vi "Database.SaveResults2.vi"(7 "Idx":i32, 8 "error in (no error)":errorcluster, 9 "Sets":T1, 10 "Data to export":T2, 11 "dbHandle":i32) -> (0 "error out":errorcluster, 1 "Export Time":timestamp, 2 "Data exported":T2, 3 "dbHandle out":i32)   [LabVIEW 2016]
uses:
  Cache/Cache.TestSteps.Fglb.ResultData.ctl
  ProdaNG/Controls/ProdaNG.ProcessResult.ctl
  ProdaNG/Controls/ProdaNG.ProcessStepResult.ctl
  ProdaNG/Controls/ProdaNG.TestStepResult.ctl
  ProdaNG/Controls/ProdaNG.TestValueResult.ctl
  Database.Data.Sets.ctl
  Tools/Translator/Translator.Message.ctl
  Tools/EventLog/EventLog.EventSource.ctl
  ProdaNG/Controls/ProdaNG.Product.ctl
  Tools/EventLog/EventLog.New(array).vi
  Tools/EventLog/EventLog.File.ReadWrite.vi
  Tools/EventLog/EventLog.Buffer.vi
  Global/ApplicationGlobal.vi
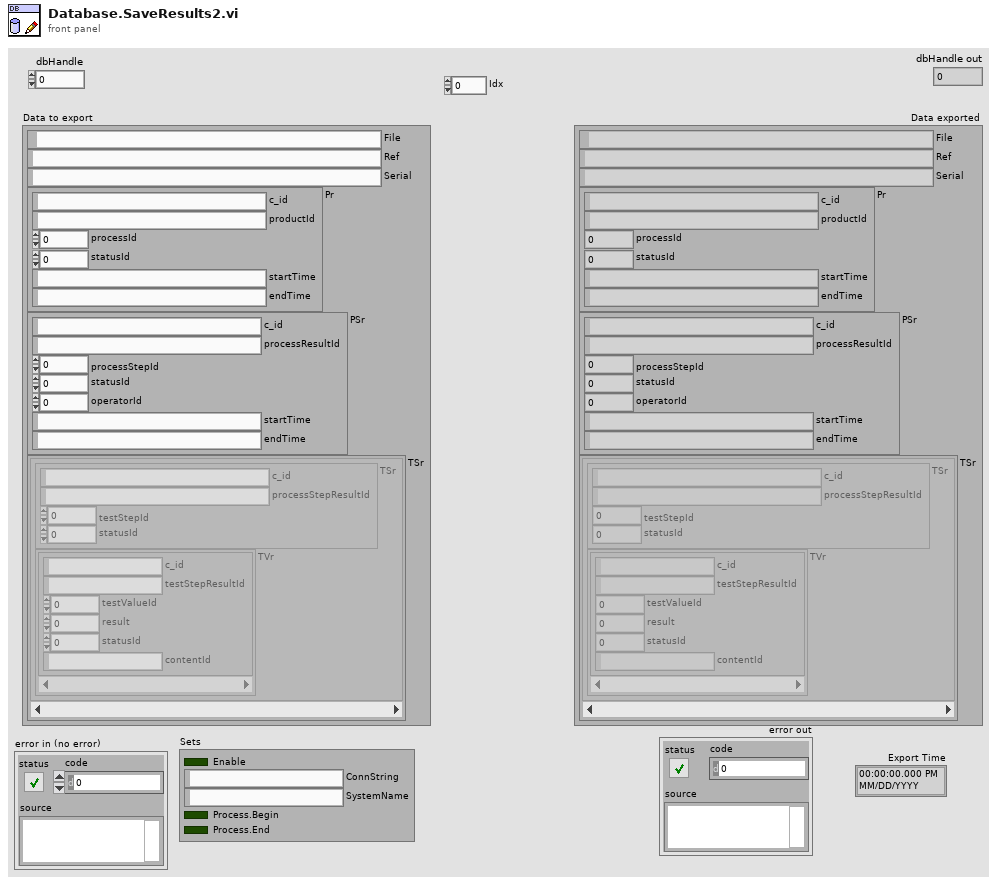
[diagram p1: front panel]
types:
  T1 = typedef "Database.Data.Sets.ctl" = cluster{"Enable":bool, "ConnString":string, "SystemName":string, "Process.Begin":bool, "Process.End":bool}
  T2 = typedef "Cache.TestSteps.Fglb.ResultData.ctl" = cluster{"File":path, "Ref":string, "Serial":string, "Pr":T3, "PSr":T4, "TSr":cluster{"TSr":T5, "TVr":T6[]}[]}
  T3 = typedef "ProdaNG.ProcessResult.ctl" = cluster{"c_id":string, "productId":string, "processId":i32, "statusId":i32, "startTime":string, "endTime":string}
  T4 = typedef "ProdaNG.ProcessStepResult.ctl" = cluster{"c_id":string, "processResultId":string, "processStepId":i32, "statusId":i32, "operatorId":i32, "startTime":string, "endTime":string}
  T5 = typedef "ProdaNG.TestStepResult.ctl" = cluster{"c_id":string, "processStepResultId":string, "testStepId":i32, "statusId":i32}
  T6 = typedef "ProdaNG.TestValueResult.ctl" = cluster{"c_id":string, "testStepResultId":string, "testValueId":i32, "result":dbl, "statusId":i32, "contentId":string}
  T7 = typedef "EventLog.EventSource.ctl" = enum16{"All", "Gui", "Cache", "PLC1", "PLC2", "PLC3", "DB", "DB01", "DB02", "DB03", "DB04", "DB05", "DB06", "DB07", "DB08", "DB09", "DB10", "DB11", "DB12", "DB13", "DB14", "DB15", "DB16"}
  T8 = typedef "Translator.Message.ctl" = enum16{"-", "Event confirmed", "Log out", "Log in", "Shutdown", "Cancel", "Start", "Continue", "Stop", "On", "Off", "OK", "NOK", "NOK %s", "This", "Prev", "Home", "Work", "In progress...", "Missing", "Empty", "Hardware failure", "Initial", "Error %d >> %s", "Error %d >> %s >> %s", "Starting %s", "Quitting %s", "Configured", "Initializing", "Quitting", "Loading", "Running %s", "Stopped", "Summary", "Do you want to continue?", "Do you want to exit?", "Log out?", "System", "All", "IDLE", "Translating...%s", "Not found", "Alarm %s", "Run", "Skip", "Abort", "Repeat", "Please wait...", "Database disconnected", "Login to database successful", "Login to database failed: %d; %s", "Get process step data for %s", "Changeover off", "Changeover into %s", "Product %s | %s found in cache with status %d at previous station", "Product %s | %s found in database with status %d at previous station", "Product %s | %s not found in cache at previous station", "Product %s | %s not found in database at previous station", "Product %s | %s found in cache with status %d at this station (%d repetion)", "Product %s | %s found in database with status %d at this station (%d repetition)", "Product %s | %s not found in cache at this station", "Product %s | %s not found in database at this station", "Product %s | %s found in cache for component %s | %s", "Product %s | %s found in database for component %s | %s", "Product not found in cache for component %s | %s", "Product not found in database for component %s | %s", "Product %s | %s connected with component %s | %s (cache)", "Product %s | %s connected with component %s | %s (database)", "New data for %s | %s (cache)", "New data for %s | %s (database)", "File %s moved (cache)", "File %s deleted (cache)", "Msg %d >> %s", "PLC LifeBit Failure", "Reconnecting DB", "Reconnecting PLC", "Free disk space is below 1GB - contact technician"}
  T9 = typedef "ProdaNG.Product.ctl" = cluster{"c_id":string, "wabcoPartId":i32, "serialNumber":string, "comment":string, "individual":i32, "crProcessStepId":i32, "mdProcessStepId":i32, "crTime":string, "mdTime":string}
  T10 = typedef "ProdaNG.Identification.ctl" = cluster{"processId":i32, "systemId":i32, "processStepId":i32, "wabcoPartId":i32}
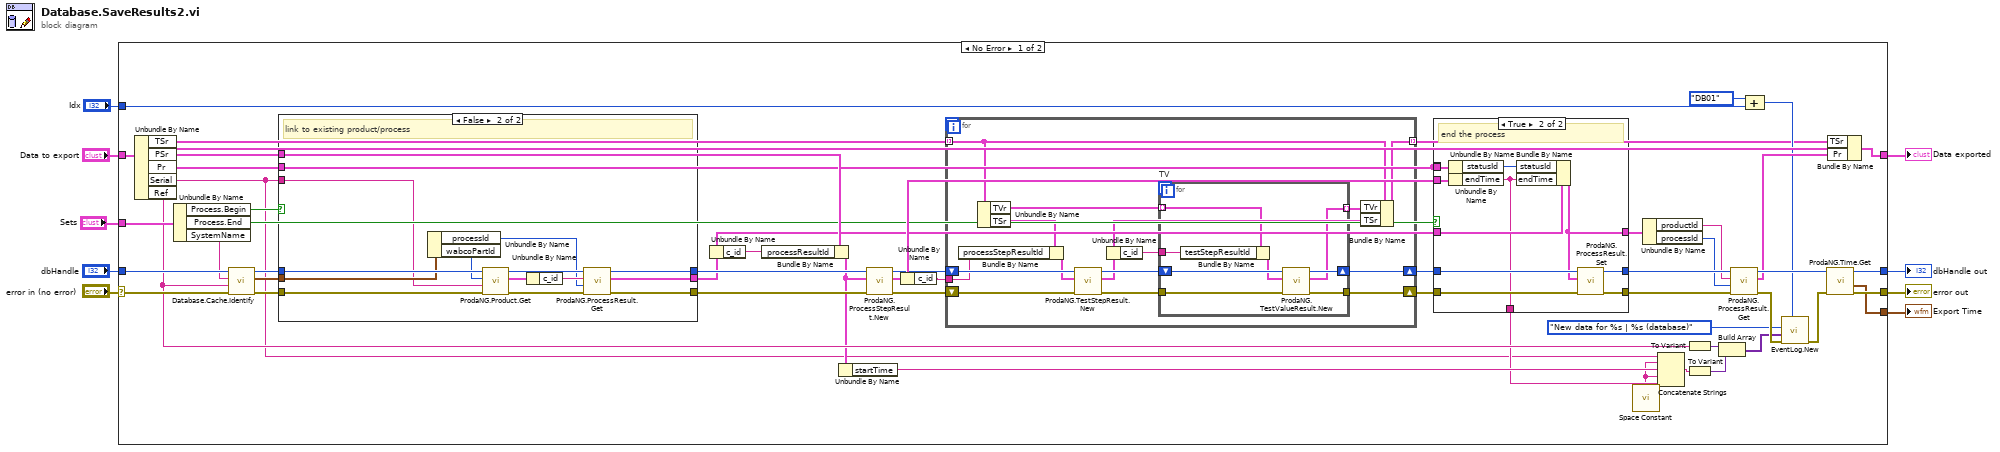
[diagram p0: block diagram]
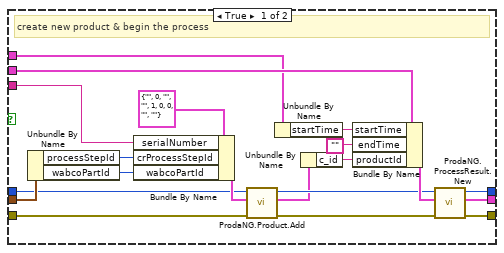
[diagram p2: hidden frame]
diagram:
  n1 = case shown="No Error" "error in (no error)" {
    selector: "error in (no error)" -> [w38 w132]
    tunnel: [w59 w132] -> w9
    tunnel: [w58 w131] -> w7
    tunnel: "dbHandle" -> [w37 w131]
    tunnel: [w57 _] -> w5
    tunnel: "Data to export" -> [w42 w130]
    tunnel: [w43 w130] -> w3
    tunnel: "Sets" -> [w40 _]
    tunnel: "Idx" -> [w30 _]
    frame No Error {
      n2 = Unbundle By Name(w42) -> ("TSr"=w28:cluster{"TSr":T5, "TVr":T6[]}[], "PSr"=w41:T4, "Pr"=w10:T3, "Serial"=w13:string, "Ref"=w29:string)
      n3 = Unbundle By Name(w40) -> ("Process.Begin"=w39:bool, "Process.End"=w25:bool, "SystemName"=w36:string)
      n4 = call "Database.Cache.Identify.vi"("error in (no error)"=w38, "Variant"=w29, "SystemName"=w36, "DB Handle in"=w37) -> ("error out"=w15:errorcluster, "SytemID"=w16:T10, "DB Handle out"=w14:i32)  [unwired: 5 in]
      n5 = case shown="False" w39 {
        tunnel: w14 -> [w90 w112]
        tunnel: w15 -> [w91 w110]
        tunnel: w10 -> [w103 _]
        tunnel: [w101 w116] -> w55
        tunnel: [w100 w114] -> w56
        tunnel: [w99 w115] -> w12
        tunnel: w41 -> [w95 _]
        tunnel: w16 -> [w92 w107]
        tunnel: w13 -> [w84 w104]
        frame True {
          # "create new product & begin the process"
          n6 = Unbundle By Name(w92) -> ("processStepId"=w86:i32, "wabcoPartId"=w85:i32)
          n7 = Bundle By Name(cluster=T9 {"c_id"="", "wabcoPartId"=0, "serialNumber"="", "comment"="", "individual"=1, "crProcessStepId"=0, "mdProcessStepId"=0, "crTime"="", "mdTime"=""} ("Product"), "serialNumber"=w84, "crProcessStepId"=w86, "wabcoPartId"=w85) -> (w93:T9)
          n8 = call "ProdaNG.Product.Add.vi"("error in (no error)"=w91, "Product"=w93, "dbHandle"=w90) -> ("error out"=w88:errorcluster, "Product out"=w87:T9, "dbHandle"=w89:i32)  [unwired: 6 in]
          n9 = Unbundle By Name(w95) -> ("startTime"=w96:string)
          n10 = Unbundle By Name(w87) -> ("c_id"=w98:string)
          n11 = Bundle By Name(cluster=w103, "startTime"=w96, "endTime"="", "productId"=w98) -> (w102:T3)
          n12 = call "ProdaNG.ProcessResult.New.vi"("error in (no error)"=w88, "ProcessResult"=w102, "dbHandle"=w89) -> ("error out"=w101:errorcluster, "ProcessResult out"=w99:T3, "dbHandle"=w100:i32)  [unwired: 6 in]
        }
        frame False {
          # "link to existing product/process"
          n13 = Unbundle By Name(w107) -> ("processId"=w105:i32, "wabcoPartId"=w106:i32)
          n14 = call "ProdaNG.Product.Get.vi"("error in (no error)"=w110, "serialNumber"=w104, "wabcoPartId"=w106, "dbHandle"=w112) -> ("error out"=w109:errorcluster, "Product"=w108:T9, "dbHandle out"=w111:i32)  [unwired: 4 in, 1 out]
          n15 = Unbundle By Name(w108) -> ("c_id"=w113:string)
          n16 = call "ProdaNG.ProcessResult.Get.vi"("error in (no error)"=w109, "processId"=w105, "productId"=w113, "dbHandle"=w111) -> ("error out"=w116:errorcluster, "ProcessResult"=w115:T3, "dbHandle out"=w114:i32)  [unwired: 4 in, 1 out]
        }
      }
      n17 = Unbundle By Name(w12) -> ("c_id"=w48:string)
      n18 = Bundle By Name(cluster=w41, "processResultId"=w48) -> (w24:T4)
      n19 = Unbundle By Name(w24) -> ("startTime"=w23:string)
      n20 = call "ProdaNG.ProcessStepResult.New.vi"("error in (no error)"=w55, "ProcessStepResult"=w24, "dbHandle"=w56) -> ("error out"=w52:errorcluster, "ProcessStepResult out"=w54:T4, "dbHandle"=w53:i32)  [unwired: 6 in]
      n21 = Unbundle By Name(w54) -> ("c_id"=w60:string)
      n22 = for "TS" {
        tunnel: w60 -> [w69]
        shift-right: [w65] -> w27
        shift-left: w53 -> [w74]
        tunnel: w28 -> [w64] mode=indexing
        shift-right: [w67] -> w26
        shift-left: w52 -> [w75]
        tunnel: [w61] -> w11 mode=indexing
        n23 = Unbundle By Name(w64) -> ("TVr"=w73:T6[], "TSr"=w66:T5)
        n24 = Bundle By Name(cluster=w66, "processStepResultId"=w69) -> (w68:T5)
        n25 = call "ProdaNG.TestStepResult.New.vi"("error in (no error)"=w75, "TestStepResult"=w68, "dbHandle"=w74) -> ("error out"=w71:errorcluster, "TestStepResult out"=w62:T5, "dbHandle"=w72:i32)  [unwired: 6 in]
        n26 = Unbundle By Name(w62) -> ("c_id"=w70:string)
        n27 = for "TV" {
          tunnel: w71 -> [w83]
          tunnel: [w78] -> w67
          tunnel: w70 -> [w80]
          tunnel: w73 -> [w81] mode=indexing
          shift-right: [w77] -> w65
          shift-left: w72 -> [w82]
          tunnel: [w76] -> w63 mode=indexing
          n28 = Bundle By Name(cluster=w81, "testStepResultId"=w80) -> (w79:T6)
          n29 = call "ProdaNG.TestValueResult.New.vi"("error in (no error)"=w83, "TestValueResult"=w79, "dbHandle"=w82) -> ("error out"=w78:errorcluster, "TestValueResult 2"=w76:T6, "dbHandle"=w77:i32)  [unwired: 6 in]
        }
        n30 = Bundle By Name(cluster=w64, "TVr"=w63, "TSr"=w62) -> (w61:cluster{"TSr":T5, "TVr":T6[]})
      }
      n31 = case shown="True" w25 {
        tunnel: w27 -> [w119 w129]
        tunnel: w26 -> [w118 w128]
        tunnel: [w119 w124] -> w51
        tunnel: [w118 w125] -> w50
        tunnel: w12 -> [w117 w127]
        tunnel: w54 -> [_ w126]
        tunnel: [w117 w123] -> w47
        tunnel: w10 -> [_ _]
        tunnel: [_ w122] -> w22
        tunnel: w10 -> [_ w121]
        frame False {
        }
        frame True {
          # "end the process"
          n32 = Unbundle By Name(w121) -> ("statusId"=w120:i32)
          n33 = Unbundle By Name(w126) -> ("endTime"=w122:string)
          n34 = Bundle By Name(cluster=w127, "statusId"=w120, "endTime"=w122) -> (w123:T3)
          n35 = call "ProdaNG.ProcessResult.Set.vi"("error in (no error)"=w128, "ProcessResult"=w123, "dbHandle"=w129) -> ("error out"=w125:errorcluster, "dbHandle"=w124:i32)  [unwired: 7 in]
        }
      }
      n36 = call <vilib>:"Space Constant.vi"() -> ("String"=w21:string)
      n37 = Unbundle By Name(w47) -> ("productId"=w46:string, "processId"=w45:i32)
      n38 = Concatenate Strings(w13, w21, w23, w21, w22) -> (w19:string)
      n39 = To Variant(anything=w29) -> (Variant=w35:variant)
      n40 = To Variant(anything=w19) -> (Variant=w18:variant)
      n41 = Build Array(w35, w18) -> (w17:variant[])
      n42 = call "ProdaNG.ProcessResult.Get.vi"("error in (no error)"=w50, "processId"=w45, "productId"=w46, "dbHandle"=w51) -> ("error out"=w32:errorcluster, "ProcessResult"=w44:T3, "dbHandle out"=w49:i32)  [unwired: 4 in, 1 out]
      n43 = Compound Arithmetic op=ADD(EventLog.EventSource."DB01" ("Source (All)"), w30) -> (w33:i32)
      n44 = call-poly "EventLog.New.vi"("Source (All)"=w33, "error in (no error)"=w32, "Arguments"=w17, "Message (-)"=Translator.Message."New data for %s | %s (database)") -> ("error out"=w31:errorcluster)  [unwired: 6 in, 1 out]
      n45 = call "ProdaNG.Time.Get.vi"("error in"=w31, "dbHandleIn"=w49) -> ("error out"=w59:errorcluster, "time"=w57:timestamp, "dbHandle"=w58:i32)  [unwired: 5 in, 1 out]
      n46 = Bundle By Name(cluster=w42, "TSr"=w11, "Pr"=w44) -> (w43:T2)
    }
    frame Error {
    }
  }
  "error out" <- w9
  "dbHandle out" <- w7
  "Export Time" <- w5
  "Data exported" <- w3
